vi "온도 센서 초기 설정.vi"(11 "클러스터":T1={"minimum value "=0.0, "maximum value "=100.0, "thermocouple type "=10072, "physical channels "=""} {"thermocouple type" items=["J"=10072, "K"=10073, "N"=10077, "R"=10082, "S"=10085, "T"=10086, "B"=10047, "E"=10055]}) -> (3 "출력 클러스터":T1)   [LabVIEW 2022 SP3]
panel:
  in  "physical channels":tag
  in  "thermocouple type":i32(ring)=10072 items=["J"=10072, "K"=10073, "N"=10077, "R"=10082, "S"=10085, "T"=10086, "B"=10047, "E"=10055]
  in  "maximum value":dbl=100.0
  in  "minimum value":dbl
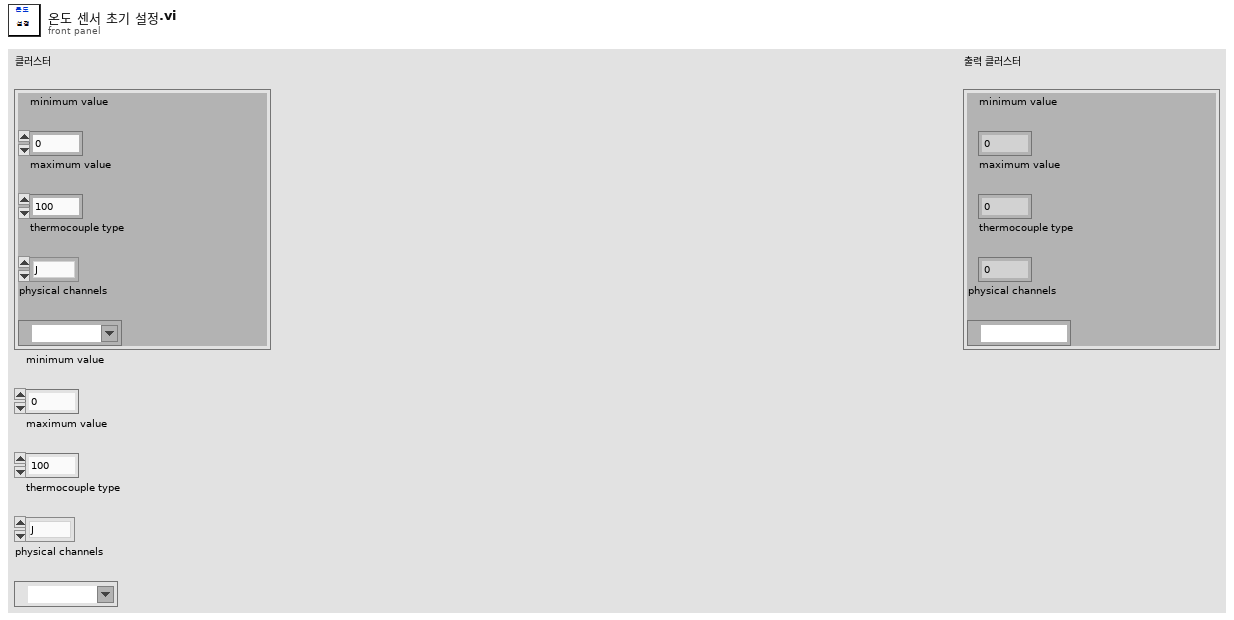
[diagram p1: front panel]
types:
  T1 = cluster{"minimum value ":dbl, "maximum value ":dbl, "thermocouple type ":i32, "physical channels ":tag}
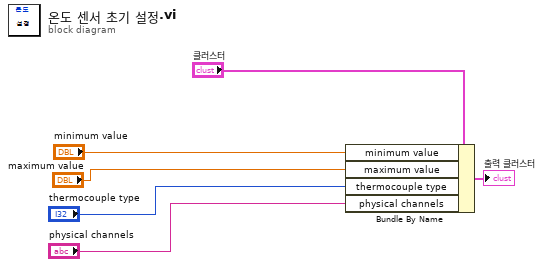
[diagram p0: block diagram]
diagram:
  n1 = Bundle By Name(cluster="클러스터", "minimum value"="minimum value", "maximum value"="maximum value", "thermocouple type"="thermocouple type", "physical channels"="physical channels") -> (→"출력 클러스터":T1)
